vi "niFpgaGenerateCode_MappingGlobal.vi"() -> ()   [LabVIEW 2017]
uses:
  <vilib>/rvi/CDR/niFpgaGenerateCode_NodeMaps.ctl
  <vilib>/rvi/CDR/niFpgaGenerateCode_NodeMap.ctl
  <vilib>/rvi/ClientSDK/Core/ErrorReporting/Public/ObjectIDHandling/nirviResholderInfo.ctl
panel:
  in  "Node Maps":T1
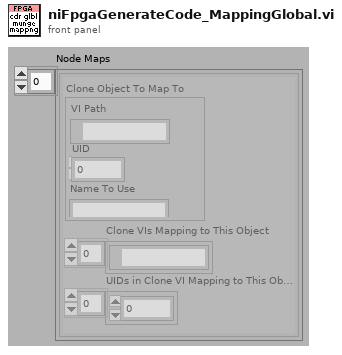
[diagram p1: front panel]
types:
  T1 = typedef "niFpgaGenerateCode_NodeMaps.ctl" = T2[]
  T2 = typedef "niFpgaGenerateCode_NodeMap.ctl" = cluster{"Clone VIs Mapping to This Object":path[], "UIDs in Clone VI Mapping to This Object":i32[], "Clone Object To Map To":T3}
  T3 = typedef "nirviResholderInfo.ctl" = cluster{"VI Path":path, "UID":u32, "Name To Use":string}
diagram:
